vi "SwitchSidesToDrawField.vi"(8 "Lado":enum16{"Esquerdo", "Direito"}(ring), 9 "enemy_robots":T2[](array[typedef]), 10 "balls":T1[](array[typedef]), 11 "our_robots":T2[](array[typedef])) -> (1 "enemy_robots switched":T2[](array[typedef]), 2 "balls switched":T1[](array[typedef]), 3 "our_robots switched":T2[](array[typedef]))   [LabVIEW 2018]
uses:
  Core/AI Robot.ctl
  Intel/Functions Enum.ctl
  Intel/AttackerStates.ctl
  Path Planning/RRT/PathDests.ctl
  Path Planning/RRT/PathDest.ctl
  Core/AI Ball.ctl
  <vilib>/Analysis/coordinate.llb/Wrap Angle (scalar).vi
  <vilib>/Analysis/NI_AAL_Angle.lvlib
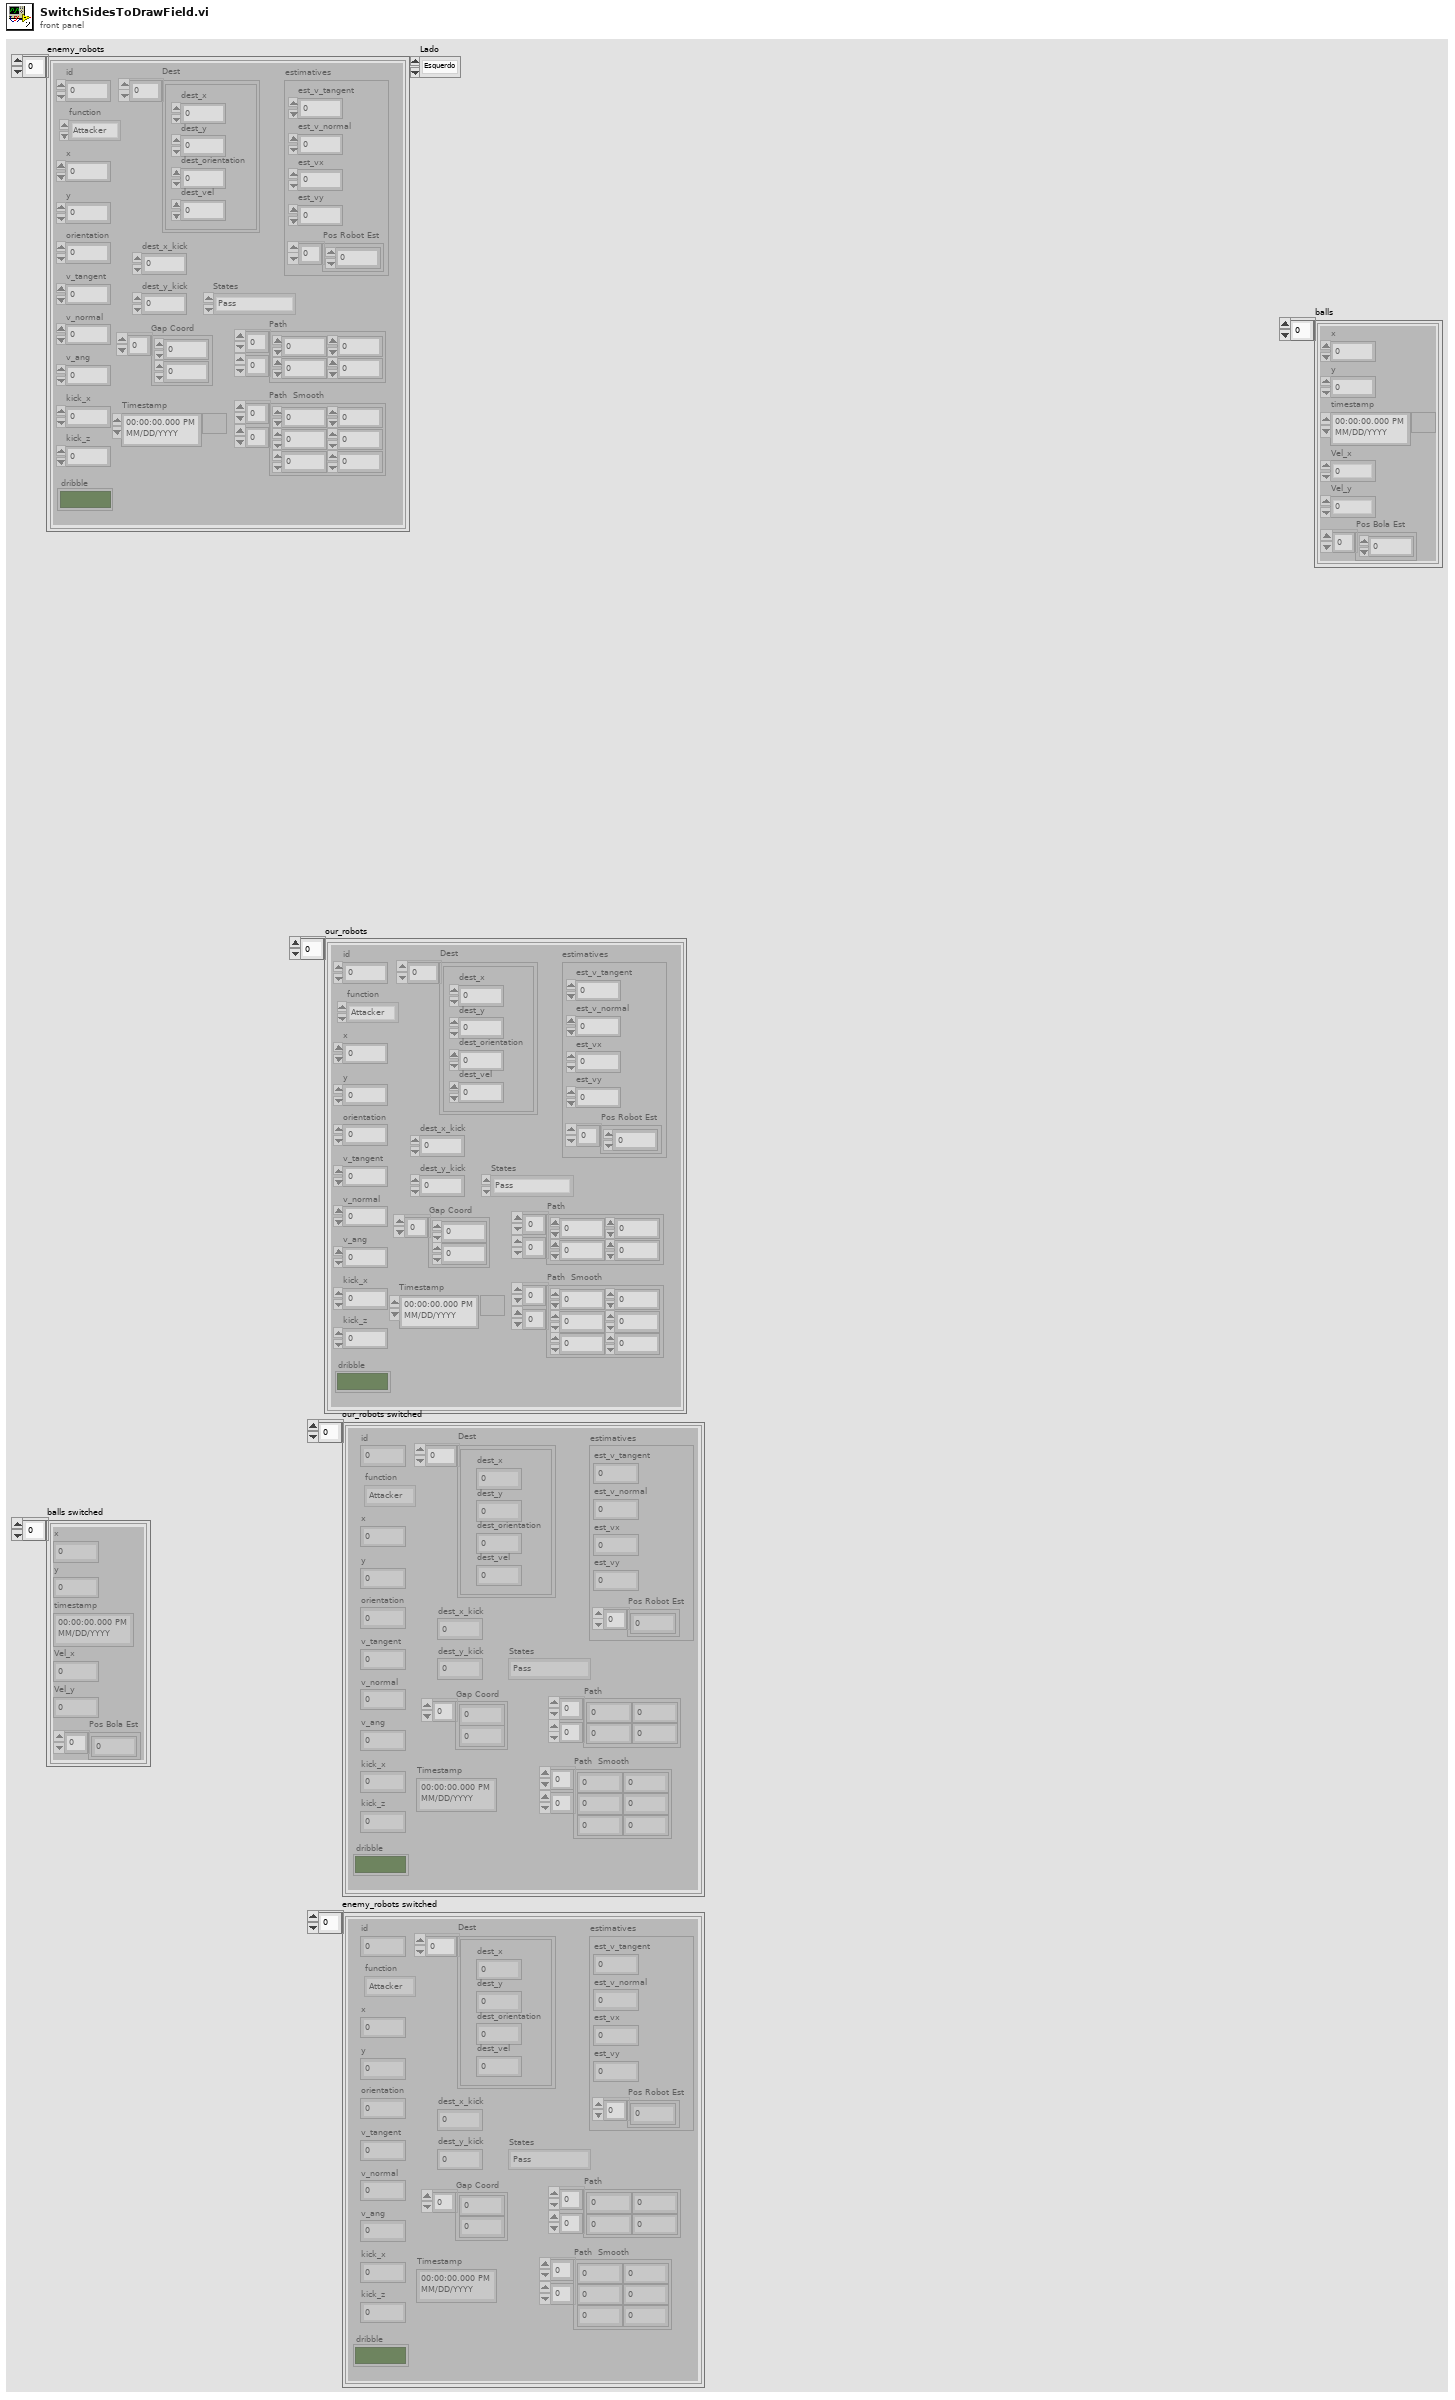
[diagram p1: front panel]
types:
  T1 = typedef "AI Ball.ctl" = cluster{"x":dbl, "y":dbl, "timestamp":timestamp, "Vel_x":dbl, "Vel_y":dbl, "Pos Bola Est":dbl[]}
  T2 = typedef "AI Robot.ctl" = cluster{"id":u32, "function":T3, "x":dbl, "y":dbl, "orientation":dbl, "v_tangent":dbl, "v_normal":dbl, "v_ang":dbl, "kick_x":dbl, "kick_z":dbl, "dribble":bool, "Timestamp":timestamp, "estimatives":cluster{"est_v_tangent":dbl, "est_v_normal":dbl, "est_vx":dbl, "est_vy":dbl, "Pos Robot Est":dbl[]}, "dest_x_kick":dbl, "dest_y_kick":dbl, "Gap Coord":dbl[], "States":T4, "Path ":dbl[][], "Path  Smooth":dbl[][], "Dest":T5}
  T3 = typedef "Functions Enum.ctl" = enum16{"Attacker", "Goalie", "Defender", "Striker", "Goto 0", "Dummy", "Kicker", "ZigZag"}
  T4 = typedef "AttackerStates.ctl" = enum16{"Pass", "GoToTangent", "BallGetting", "GoToKick", "Rotate anti-clockwise", "Rotate Clockwise", ""}
  T5 = typedef "PathDests.ctl" = T6[]
  T6 = typedef "PathDest.ctl" = cluster{"dest_x":dbl, "dest_y":dbl, "dest_orientation":dbl, "dest_vel":dbl}
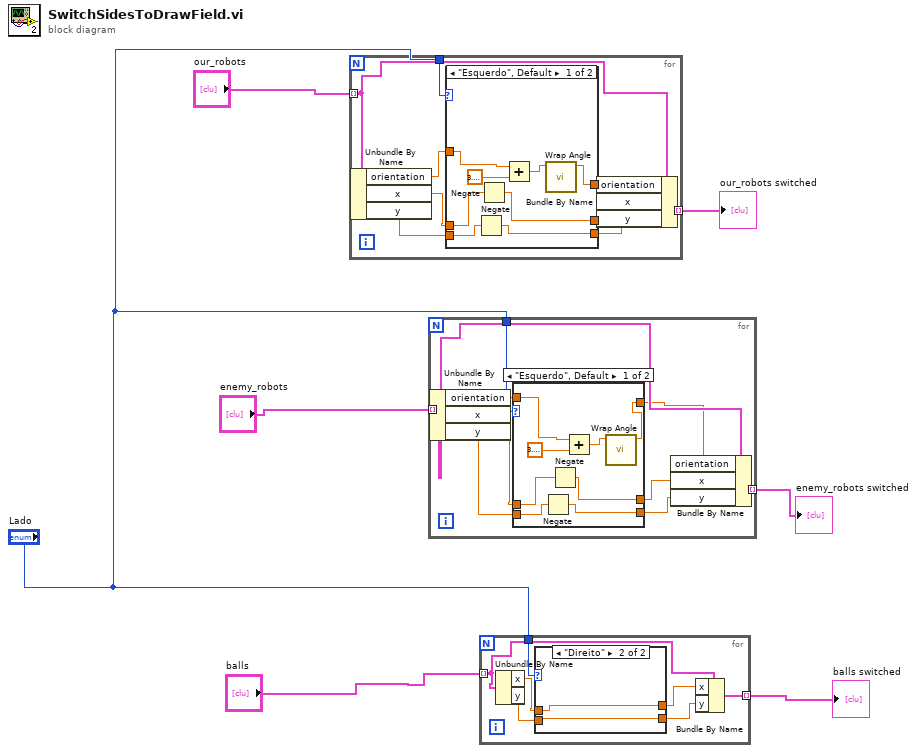
[diagram p0: block diagram]
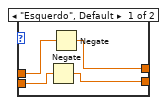
[diagram p4: hidden frame]
diagram:
  n1 = for {
    tunnel: "our_robots" -> [w15] mode=indexing
    tunnel: [w16] -> w4 mode=indexing
    tunnel: "Lado" -> [w14]
    n2 = Unbundle By Name(w15) -> ("orientation"=w9:dbl, "x"=w13:dbl, "y"=w12:dbl)
    n3 = case shown="\"Esquerdo\", Default" w14 {
      tunnel: w13 -> [w24 w27]
      tunnel: w12 -> [w23 w26]
      tunnel: [w22 w27] -> w11
      tunnel: [w21 w26] -> w10
      tunnel: w9 -> [w18 w25]
      tunnel: [w17 w25] -> w8
      frame "Esquerdo", Default {
        n4 = Negate(x=w23) -> (-x=w21:dbl)
        n5 = Negate(x=w24) -> (-x=w22:dbl)
        n6 = Add(x=w18, y=3.141592653589793) -> (x+y=w19:dbl)
        n7 = call-poly <vilib>:"Wrap Angle.vi"("angle in"=w19) -> ("angle out"=w17:dbl)  [unwired: 9 in, 1 out]
      }
      frame "Direito" {
      }
    }
    n8 = Bundle By Name(cluster=w15, "orientation"=w8, "x"=w11, "y"=w10) -> (w16:T2)
  }
  "our_robots switched" <- w4
  n9 = for {
    tunnel: "enemy_robots" -> [w35] mode=indexing
    tunnel: [w36] -> w3 mode=indexing
    tunnel: "Lado" -> [w34]
    n10 = Unbundle By Name(w35) -> ("orientation"=w28:dbl, "x"=w33:dbl, "y"=w32:dbl)
    n11 = case shown="\"Esquerdo\", Default" w34 {
      tunnel: w33 -> [w44 w47]
      tunnel: w32 -> [w43 w46]
      tunnel: [w42 w47] -> w31
      tunnel: [w41 w46] -> w30
      tunnel: [w37 w45] -> w29
      tunnel: w28 -> [w38 w45]
      frame "Esquerdo", Default {
        n12 = Negate(x=w43) -> (-x=w41:dbl)
        n13 = Negate(x=w44) -> (-x=w42:dbl)
        n14 = Add(x=w38, y=3.141592653589793) -> (x+y=w39:dbl)
        n15 = call-poly <vilib>:"Wrap Angle.vi"("angle in"=w39) -> ("angle out"=w37:dbl)  [unwired: 9 in, 1 out]
      }
      frame "Direito" {
      }
    }
    n16 = Bundle By Name(cluster=w35, "orientation"=w29, "x"=w31, "y"=w30) -> (w36:T2)
  }
  "enemy_robots switched" <- w3
  n17 = for {
    tunnel: "balls" -> [w53] mode=indexing
    tunnel: [w54] -> w2 mode=indexing
    tunnel: "Lado" -> [w52]
    n18 = Unbundle By Name(w53) -> ("x"=w51:dbl, "y"=w50:dbl)
    n19 = case shown="\"Direito\"" w52 {
      tunnel: w51 -> [w58 w60]
      tunnel: w50 -> [w57 w59]
      tunnel: [w56 w60] -> w49
      tunnel: [w55 w59] -> w48
      frame "Esquerdo", Default {
        n20 = Negate(x=w57) -> (-x=w55:dbl)
        n21 = Negate(x=w58) -> (-x=w56:dbl)
      }
      frame "Direito" {
      }
    }
    n22 = Bundle By Name(cluster=w53, "x"=w49, "y"=w48) -> (w54:T1)
  }
  "balls switched" <- w2
